vi "SCT.vi"(0 "System no.":i32=1 min=1 max=4 step=1, 3 "Cycle time (ms)":i16=1 min=0 max=20 step=1, 5 "error in":errorcluster) -> (14 "Controller error":bool, 19 "error out":errorcluster)   [LabVIEW 2020]
doc: "Sets cycle time for MOV!/MOV command in s. Controller error is TRUE if selected system reports an error code which is not 0.\n\nC-887, F-206, M-8X0: For GCS syntax version = GCS 1.0 (Check with CSV?.vi. If CSV?.vi is not supported, syntax version is GCS 1.0), sets cycle time for MOV! command.\nFor GCS 2.0 or higher, sets cycle time for MOV command. Parameter 0x19001900 must be set to 1 in this case (SPA.vi), see controller user manual for details."
panel:
  # "Set cycle time for MOV! command in msec."
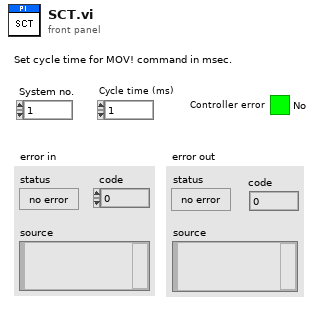
[diagram p1: front panel]
types:
  T1 = enum16{"Disable error check", "Force error check", "Use global settings"}
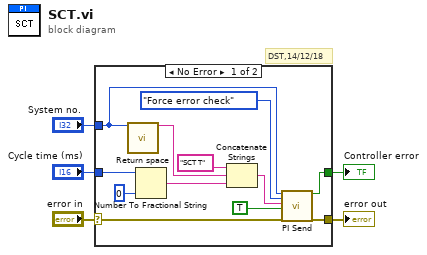
[diagram p0: block diagram]
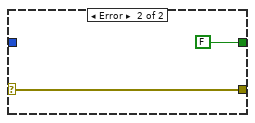
[diagram p2: hidden frame]
diagram:
  # "DST,14/12/18"
  n1 = case shown="No Error" "error in" {
    selector: "error in" -> [w6 w19]
    tunnel: "Cycle time (ms)" -> [w16 _]
    tunnel: "System no." -> [w11 _]
    tunnel: [w9 FALSE ("Controller error")] -> w3
    tunnel: [w8 w19] -> w2
    frame No Error {
      n2 = call "Return space.vi"("System no."=w11) -> ("String out"=w10:string)  [unwired: 1 in, 17 out]
      n3 = Number To Fractional String(number=w16, precision (6)=i16 0) -> (F-format string=w12:string)  [unwired: 2 out]
      n4 = Concatenate Strings("SCT T", w10, w12) -> (w13:string)
      n5 = call "PI Send.vi"("System no."=w11, "Error check settings"=T1."Force error check", "String to send"=w13, "Attach termination char.?"=TRUE ("Attach Linefeed?"), "error in"=w6) -> ("Controller error"=w9:bool, "error out"=w8:errorcluster)  [unwired: 1 in, 12 out]
    }
    frame Error {
    }
  }
  "error out" <- w2
  "Controller error" <- w3
